vi "step1 TestIfUppercrossSolved.vi"(8 "error in (no error)":errorcluster, 11 "cube in":T1) -> (0 "error out":errorcluster, 2 "uppercross solved?":bool)   [LabVIEW 2011]
uses:
  Typedef/cube.ctl
  Typedef/face.ctl
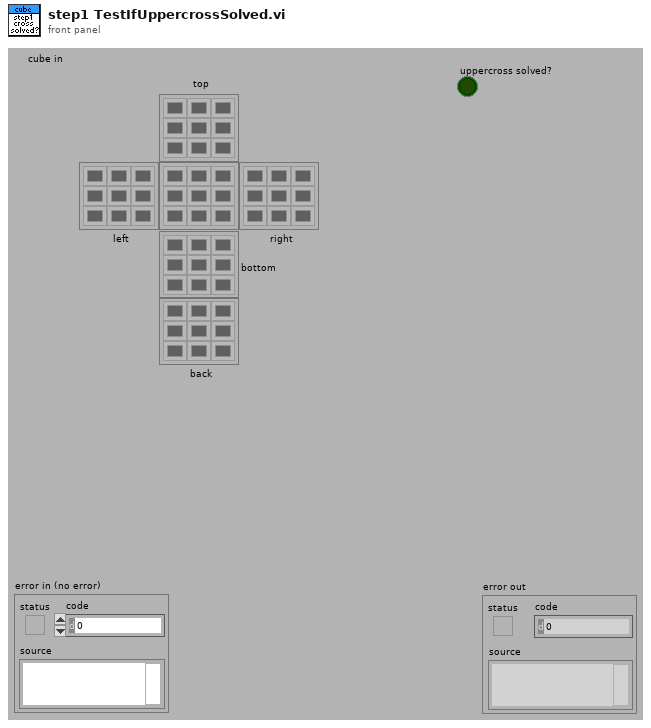
[diagram p1: front panel]
types:
  T1 = typedef "cube.ctl" = cluster{"top":T2, "left":T2, "right":T2, "bottom":T2, "back":T2, "front":T2}
  T2 = typedef "face.ctl" = u32[][]
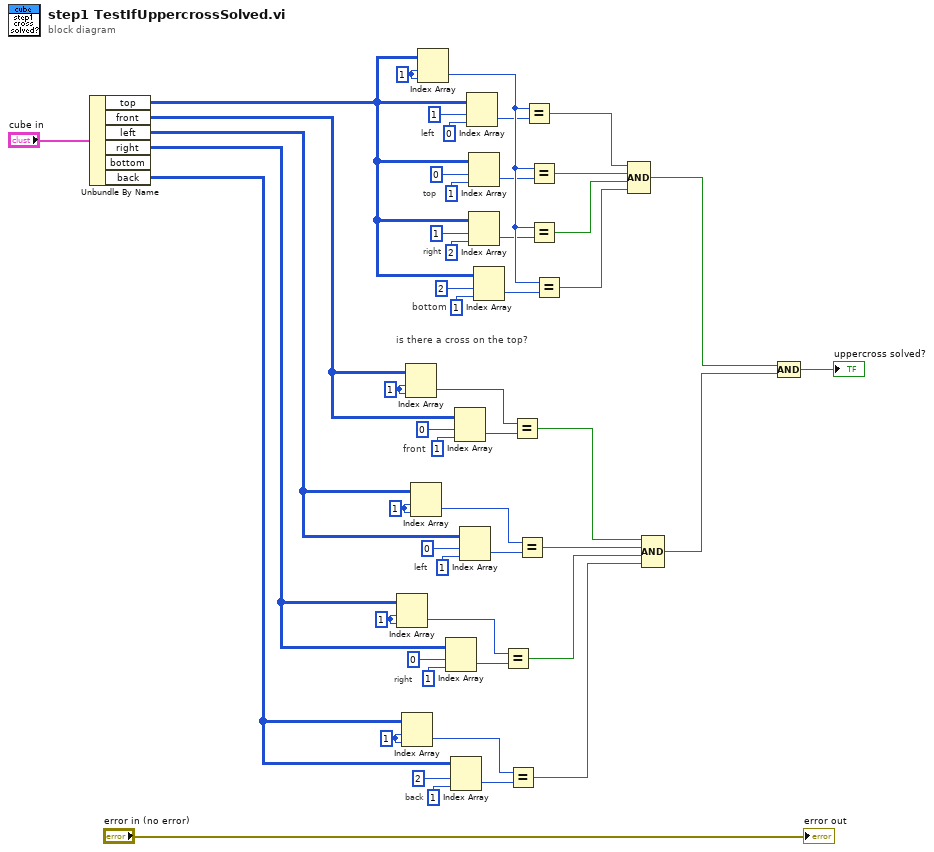
[diagram p0: block diagram]
diagram:
  w35 = 1 ("index (row)")
  w40 = 1 ("index (row)")
  w29 = 1 ("index (row)")
  w23 = 1 ("index (row)")
  w5 = 1 ("index (row)")
  # "right"
  # "back"
  # "front"
  # "left"
  # "is there a cross on the top?"
  # "bottom"
  # "right"
  # "top"
  # "left"
  n1 = Unbundle By Name("cube in") -> ("top"=w16:T2, "front"=w32:T2, "left"=w26:T2, "right"=w43:T2, "back"=w44:T2)  [unwired: 1 out]
  n2 = Index Array(array=w43, index (row)=w35, index (col)=w35) -> (element=w33:u32)
  n3 = Index Array(array=w44, index (row)=w40, index (col)=w40) -> (element=w42:u32)
  n4 = Index Array(array=w32, index (row)=w29, index (col)=w29) -> (element=w31:u32)
  n5 = Index Array(array=w26, index (row)=w23, index (col)=w23) -> (element=w21:u32)
  n6 = Index Array(array=w16, index (row)=w5, index (col)=w5) -> (element=w52:u32)
  n7 = Index Array(array=w43, index (row)=0, index (col)=1 ("disabled index (col)")) -> (element=w34:u32)
  n8 = Index Array(array=w44, index (row)=2, index (col)=1 ("disabled index (col)")) -> (element=w41:u32)
  n9 = Index Array(array=w32, index (row)=0, index (col)=1 ("disabled index (col)")) -> (element=w30:u32)
  n10 = Index Array(array=w26, index (row)=0, index (col)=1 ("disabled index (col)")) -> (element=w22:u32)
  n11 = Index Array(array=w16, index (row)=1, index (col)=0 ("disabled index (col)")) -> (element=w6:u32)
  n12 = Index Array(array=w16, index (row)=0, index (col)=1 ("disabled index (col)")) -> (element=w9:u32)
  n13 = Index Array(array=w16, index (row)=1, index (col)=2 ("disabled index (col)")) -> (element=w12:u32)
  n14 = Index Array(array=w16, index (row)=2, index (col)=1 ("disabled index (col)")) -> (element=w13:u32)
  n15 = Equal?(x=w33, y=w34) -> (x = y?=w47:bool)
  n16 = Equal?(x=w42, y=w41) -> (x = y?=w48:bool)
  n17 = Equal?(x=w31, y=w30) -> (x = y?=w45:bool)
  n18 = Equal?(x=w21, y=w22) -> (x = y?=w46:bool)
  n19 = Equal?(x=w52, y=w6) -> (x = y?=w17:bool)
  n20 = Equal?(x=w52, y=w9) -> (x = y?=w18:bool)
  n21 = Equal?(x=w52, y=w12) -> (x = y?=w19:bool)
  n22 = Equal?(x=w52, y=w13) -> (x = y?=w20:bool)
  n23 = Compound Arithmetic op=AND(w17, w18, w19, w20) -> (w49:bool)
  n24 = Compound Arithmetic op=AND(w45, w46, w47, w48) -> (w50:bool)
  n25 = Compound Arithmetic op=AND(w49, w50) -> (→"uppercross solved?":bool)
  "error out" <- "error in (no error)"
